vi "Calculate Cyclomatic Complexity.vi"(8 "error in":errorcluster, 11 "File Info in":T1) -> (0 "error out":errorcluster, 3 "File Info out":T1)   [LabVIEW 2020, in "Peer Review.lvclass"]
uses:
  Peer Review.lvclass
  TypeDefs/File Info.ctl
  TypeDefs/File State.ctl
  TypeDefs/VI Type.ctl
  <vilib>/Utility/traverseref.llb/TRef TravTarget.ctl
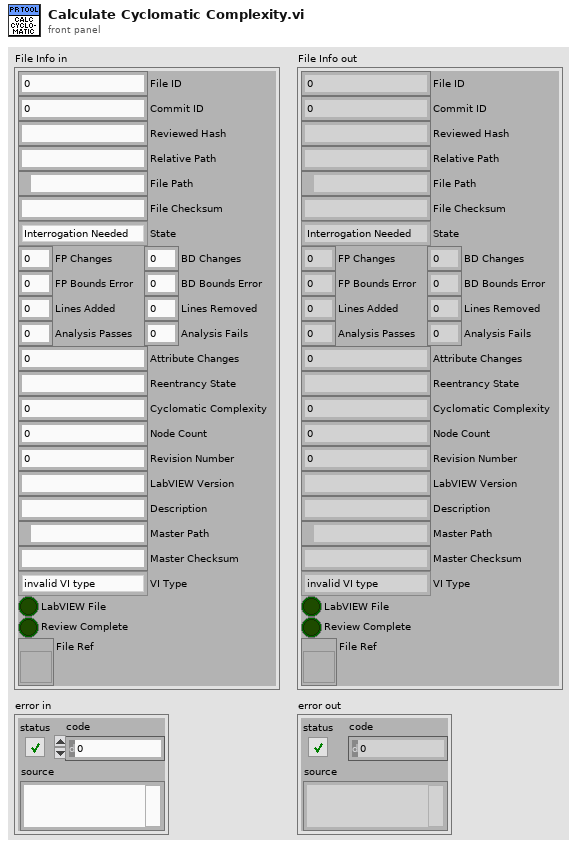
[diagram p1: front panel]
types:
  T1 = typedef "Peer Review.lvclass/File Info.ctl" = cluster{"File ID":i32, "Commit ID":i32, "Reviewed Hash":string, "Relative Path":string, "File Path":path, "File Checksum":string, "State":T2, "FP Changes":i32, "BD Changes":i32, "FP Bounds Error":dbl, "BD Bounds Error":dbl, "Lines Added":i32, "Lines Removed":i32, "Analysis Passes":i32, "Analysis Fails":i32, "Attribute Changes":i32, "Reentrancy State":string, "Cyclomatic Complexity":i32, "Node Count":i32, "Revision Number":u32, "LabVIEW Version":string, "Description":string, "Master Path":path, "Master Checksum":string, "VI Type":T3, "LabVIEW File":bool, "Review Complete":bool, "File Ref":refnum<vi>}
  T2 = typedef "Peer Review.lvclass/File State.ctl" = enum16{"Interrogation Needed", "Modified", "Deleted", "Added", "Matches Previous", "No Changes", "Moved"}
  T3 = typedef "Peer Review.lvclass/VI Type.ctl" = enum32{"invalid VI type", "Standard VI", "Control VI", "Global VI", "Polymorphic VI", "Configuration VI", "SubSystem", "Facade VI", "Method VI", "Statechart Diagram VI"}
  T4 = typedef "TRef TravTarget.ctl" = enum16{"FP", "BD", "Other"}
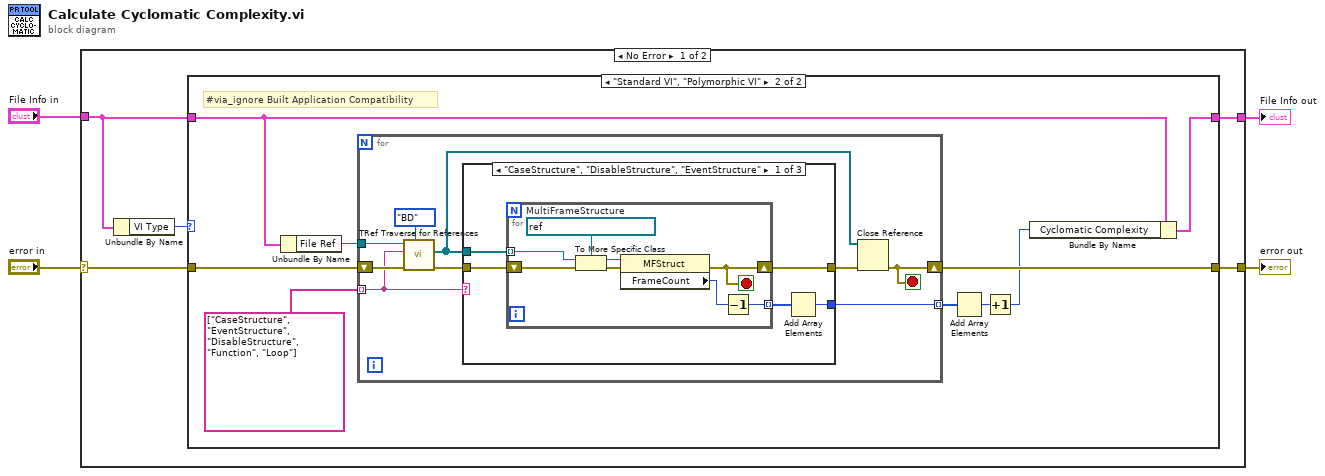
[diagram p0: block diagram]
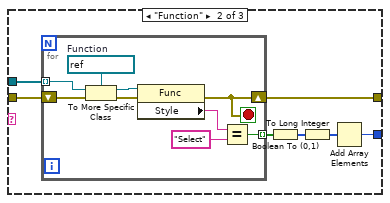
[diagram p3: hidden frame]
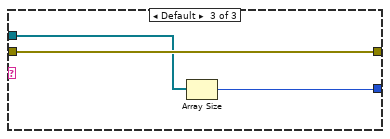
[diagram p4: hidden frame]
diagram:
  n1 = case shown="No Error" "error in" {
    selector: "error in" -> [w7 w63]
    tunnel: [w9 w63] -> w4
    tunnel: "File Info in" -> [w6 w62]
    tunnel: [w5 w62] -> w1
    frame No Error {
      n2 = Unbundle By Name(w6) -> ("VI Type"=w8:T3)
      n3 = case shown="\"Standard VI\", \"Polymorphic VI\"" w8 {
        tunnel: [w11 w18] -> w9
        tunnel: w7 -> [w11 w16]
        tunnel: w6 -> [w10 w14]
        tunnel: [w10 w12] -> w5
        frame Default {
        }
        frame "Standard VI", "Polymorphic VI" {
          # "#via_ignore Built Application Compatibility"
          n4 = Unbundle By Name(w14) -> ("File Ref"=w15:refnum<vi>)
          n5 = for {
            tunnel: string[] ["CaseStructure", "EventStructure", "DisableStructure", "Function", "Loop"] -> [w24] mode=indexing
            tunnel: [w29] -> w20 mode=indexing
            tunnel: w15 -> [w27]
            shift-right: [w21] -> w18
            shift-left: w16 -> [w28]
            stop <- w21 stop-if-true
            n6 = call <vilib>:"TRef Traverse for References.vi"("Traverse Target"=TRef_TravTarget."BD", "error in (no error)"=w28, "Class Name"=w24, "VI Refnum"=w27) -> ("error out"=w25:errorcluster, "References"=w23:refnum<vi>[])  [unwired: 1 in, 5 out]
            n7 = case shown="\"CaseStructure\", \"DisableStructure\", \"EventStructure\"" w24 {
              tunnel: [w31 w44 w61] -> w22
              tunnel: [w34 w49 w59] -> w29
              tunnel: w23 -> [w32 w45 w60]
              tunnel: w25 -> [w30 w46 w61]
              frame "CaseStructure", "DisableStructure", "EventStructure" {
                n8 = for {
                  tunnel: w32 -> [w42] mode=indexing
                  shift-right: [w35] -> w31
                  shift-left: w30 -> [w41]
                  tunnel: [w40] -> w33 mode=indexing
                  stop <- w35 stop-if-true
                  w38 = refnum<vi> refnum  # MultiFrameStructure
                  n9 = To More Specific Class(target class=w38, reference=w42, error in=w41) -> (specific class reference=w37:refnum<vi>, error out=w39:errorcluster)
                  n10 = property on="Property Node" class="MFStruct"(reference=w37, error in=w39) -> (error out=w35:errorcluster, "FrameCount"=w36:i32)  [unwired: 1 out]
                  n11 = Decrement(x=w36) -> (x-1=w40:i32)
                }
                n12 = Add Array Elements(numeric array=w33) -> (sum=w34:i32)
              }
              frame "Function" {
                n13 = for {
                  tunnel: w45 -> [w56] mode=indexing
                  shift-right: [w50] -> w44
                  shift-left: w46 -> [w54]
                  tunnel: [w51] -> w48 mode=indexing
                  stop <- w50 stop-if-true
                  w57 = refnum<vi> refnum  # Function
                  n14 = To More Specific Class(target class=w57, reference=w56, error in=w54) -> (specific class reference=w58:refnum<vi>, error out=w55:errorcluster)
                  n15 = property on="Property Node" class="Func"(reference=w58, error in=w55) -> (error out=w50:errorcluster, "Style"=w53:string)  [unwired: 1 out]
                  n16 = Equal?(x=w53, y="Select") -> (x = y?=w51:bool)
                }
                n17 = Boolean To (0,1)(Boolean=w48) -> (0, 1=w47:i16[])
                n18 = To Long Integer(number=w47) -> (32bit integer=w43:i32[])
                n19 = Add Array Elements(numeric array=w43) -> (sum=w49:i32)
              }
              frame Default {
                n20 = Array Size(array=w60) -> (size(s)=w59:i32)
              }
            }
            n21 = Close Reference(reference=w23, error in (no error)=w22) -> (error out=w21:errorcluster)
          }
          n22 = Add Array Elements(numeric array=w20) -> (sum=w19:i32)
          n23 = Increment(x=w19) -> (x+1=w13:i32)
          n24 = Bundle By Name(cluster=w14, "Cyclomatic Complexity"=w13) -> (w12:T1)
        }
      }
    }
    frame Error {
    }
  }
  "error out" <- w4
  "File Info out" <- w1
